vi "DSiam.vi"() -> ()   [LabVIEW 2011]
uses:
  SIAM/SIAM_command.ctl
  SIAM/SIAM-send.ctl
panel:
  out "notifier name":string
  out "send error":errorcluster
  out "value send":dbl
  out "Running":bool
  in  "Scales and Tickets":T1(array[cluster])=[{"ticketID"=514, "Queue/Variable"=FALSE, "name"="stage.z", "Scale"=2e-09, "Offset(HWunits)"=0.0}]
  out "address":string="10.153.70.38"
  out "remote port or service name":u16=3
  out "connect error":errorcluster
  out "Return":i32[](array[numeric]) format="%.0x"
  out "recieve error":errorcluster
  out "Connected":bool
  # "to do\nlimits?\nclosed loop über DSmartmove oder DSIAM oder Smartconnect?\n...\n...\n\n.. Objektivwechsel..."
  # "1122=normal exit"
  # "66=normal exit"
  # "bisher üblich steps/units!!! Logischer für filter!"
  # "becarefull with queues, if there is no reciever it is a memory leak"
  # "ticket  is also inside SIAM-TMSI.vi"
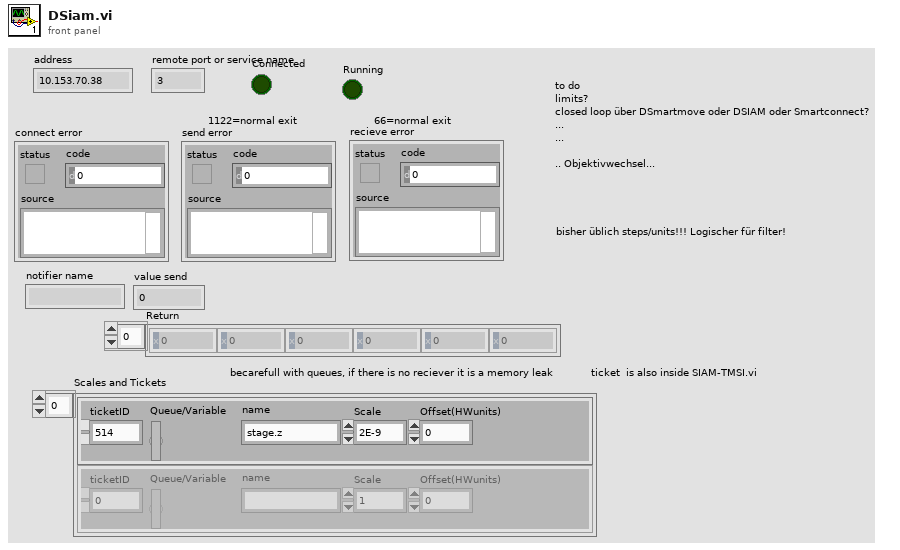
[diagram p1: front panel]
types:
  T1 = cluster{"ticketID":i32, "Queue/Variable":bool, "name":string, "Scale":dbl, "Offset(HWunits)":dbl}[]
  T2 = enum16{"None/#Datasets", "Clear", "TagValueOf#", "AddValues", "ReadValue", "ChangeValue", "Get all"}
  T3 = cluster{"Scale":dbl, "Offset(HWunits)":dbl, "ticketID":i32}[]
  T4 = typedef "SIAM-send.ctl" = enum16{"validID", "storeID", "enable", "rundirect", "sendlist", "run", "stop", "readRegister", "sendValue", "storeStatus"}
  T5 = enum8{"Ch0", "Ch1", "x-Galvo", "y-Galvo", "z-Focus"}
  T6 = enum16{"Ch0", "Ch1", "x-Galvo", "y-Galvo", "z-Focus"}
  T7 = enum16{"Standard", "Buffered", "CRLF", "Immediate"}
  T8 = typedef "SIAM_command.ctl" = u32
  T9 = cluster{"Delay 10µs":u32, "command":T8, "P0":i32, "P1":i32, "P2":i32, "P3":i32, "P4":i32, "P5-ticket":i32}
  T10 = cluster{"Scale":ext, "Offset(HWunits)":ext, "ticketID":i32}[]
  T11 = cluster{"ticketID":i32, "Queue/Variable":bool, "name":string, "Scale":dbl, "Offset(HWunits)":dbl}
  T12 = cluster{"variables":string[], cluster{"Scale":ext, "Offset(HWunits)":ext, "ticketID":i32}[]}
  T13 = cluster{"default value 2":dbl, "default value 1":dbl}
  T14 = cluster{"Delay 10µs":u32, "command":T8, "P0":i32, "P1":i32, "P2":i32, "P3":i32, "P4":i32, "P5-ticket":i32}[]
  T15 = cluster{"Scale":ext, "Offset(HWunits)":ext, "ticketID":i32}
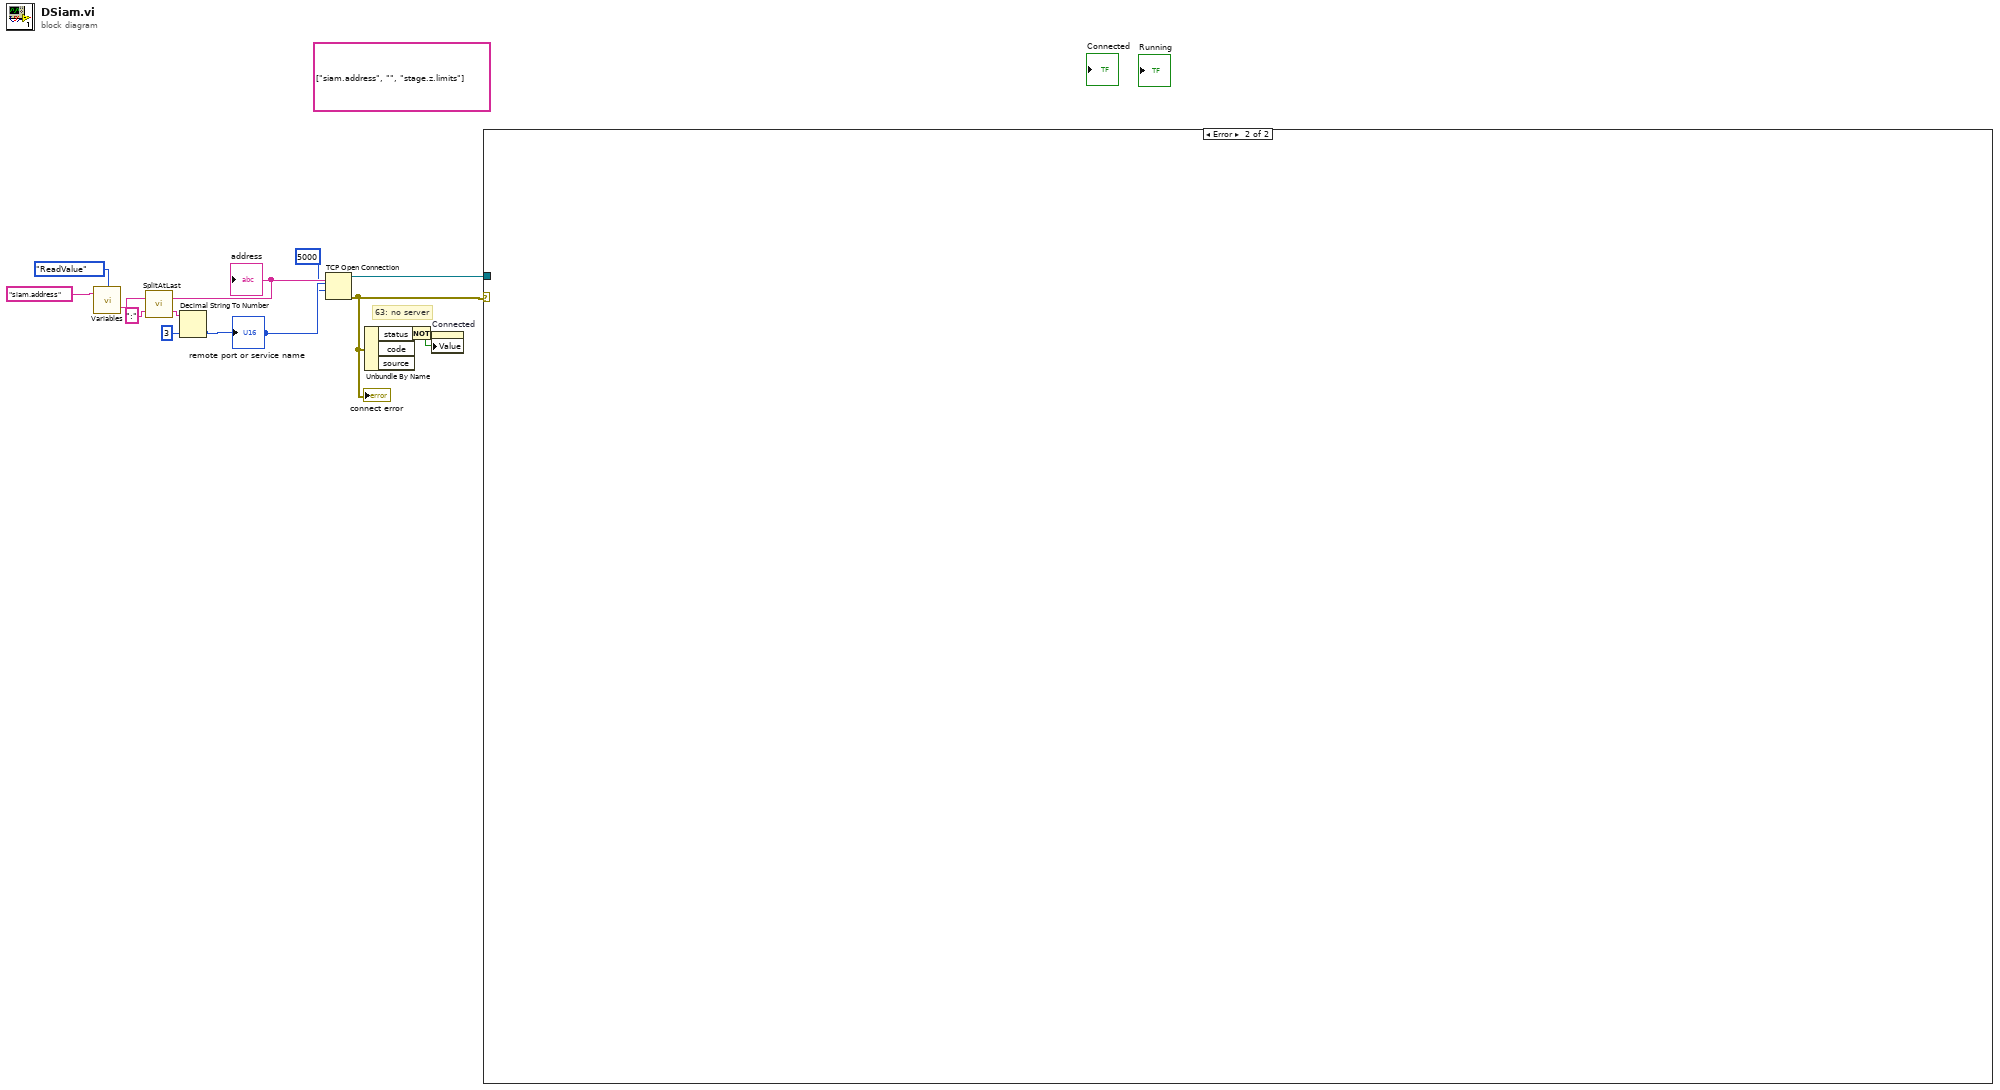
[diagram p0: block diagram]
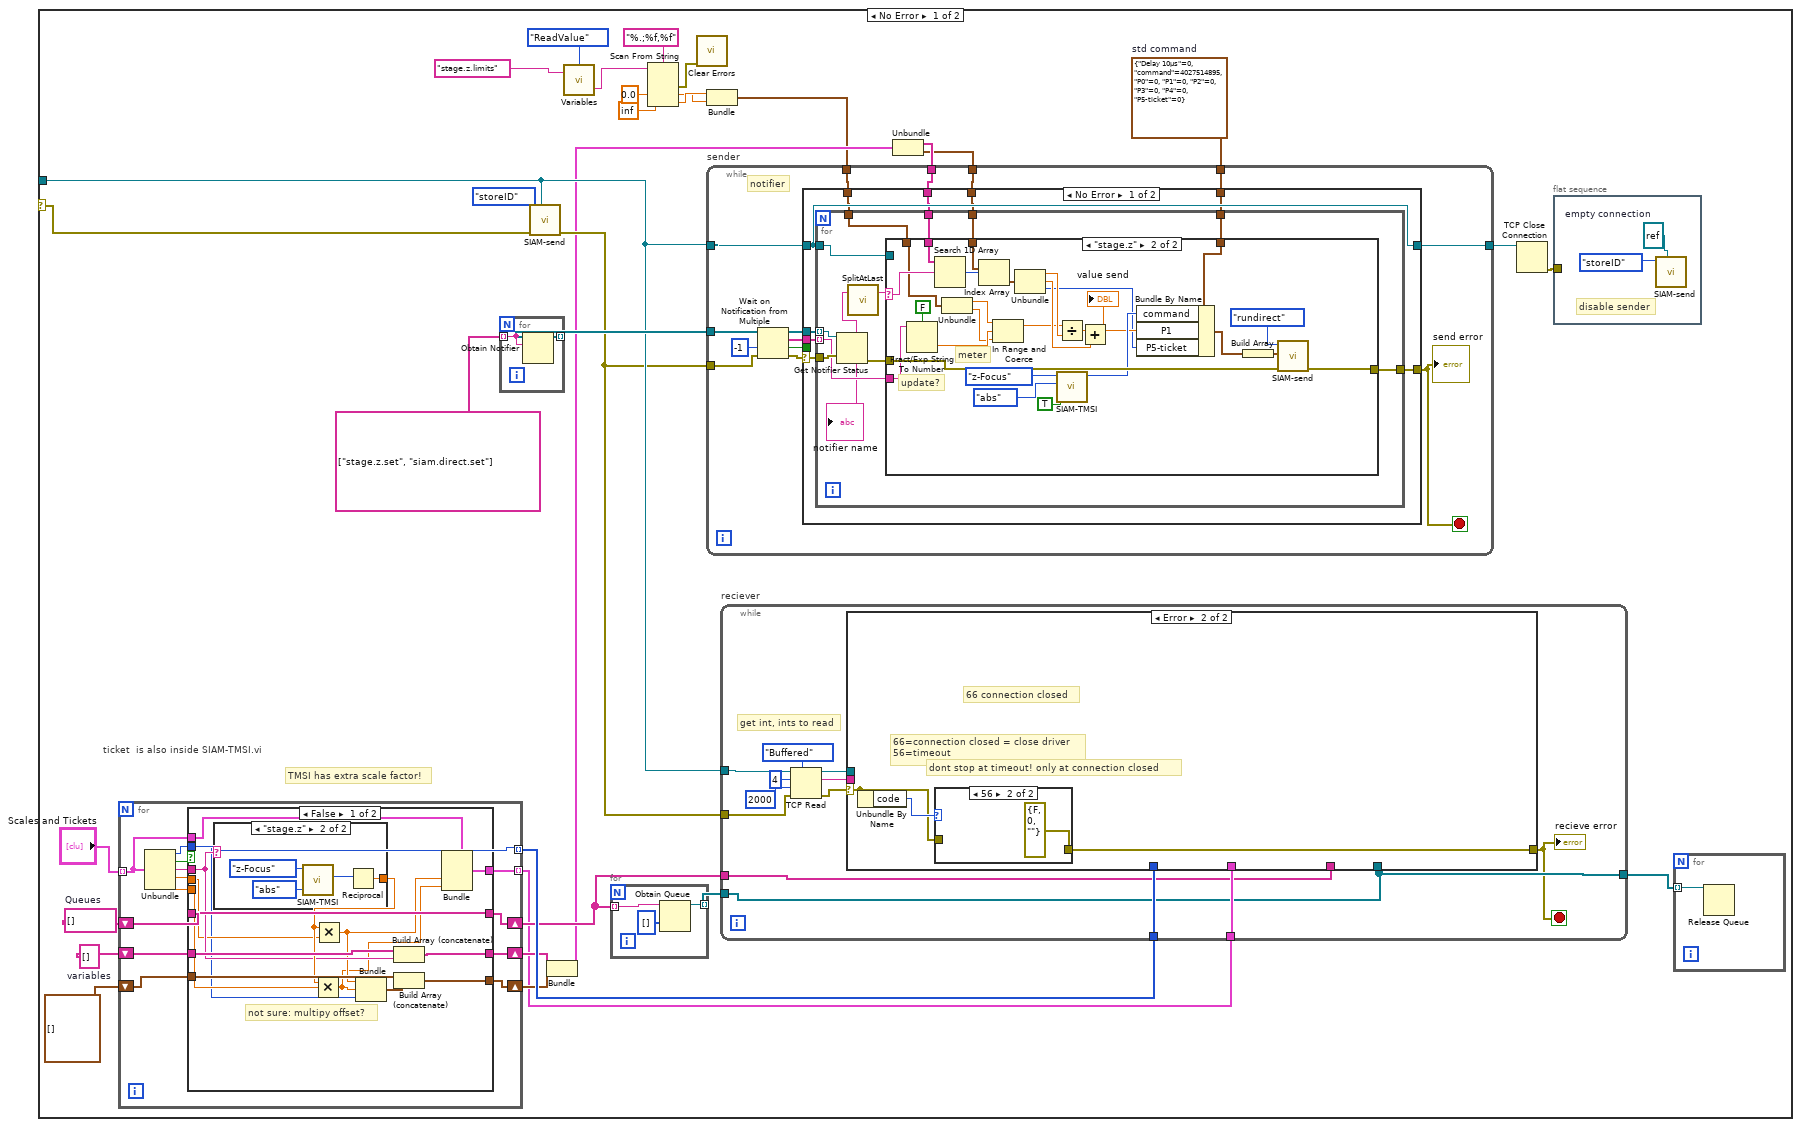
[diagram p2: hidden frame]
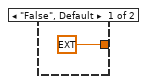
[diagram p3: hidden frame]
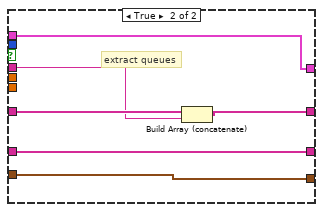
[diagram p4: hidden frame]
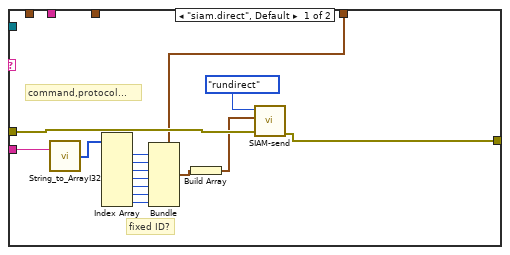
[diagram p5: hidden frame]
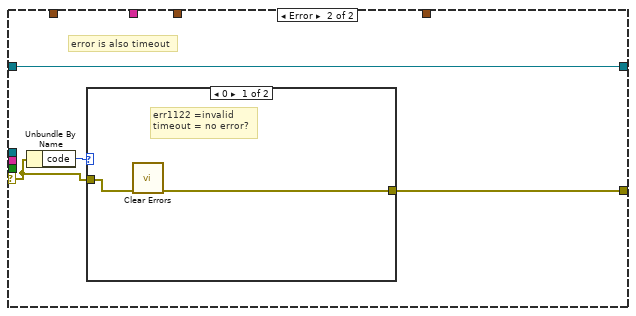
[diagram p6: hidden frame]
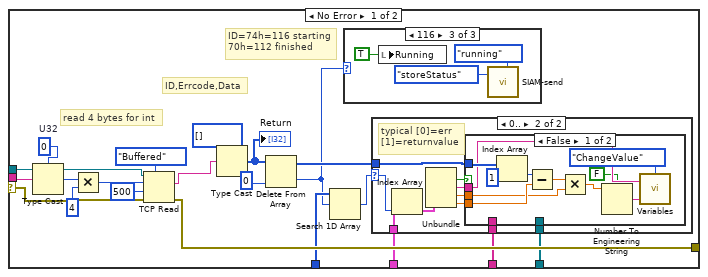
[diagram p8: hidden frame]
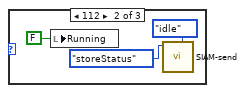
[diagram p10: hidden frame]
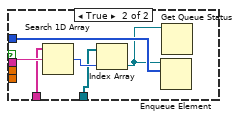
[diagram p12: hidden frame]
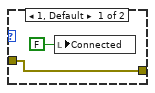
[diagram p13: hidden frame]
diagram:
  (unwired) string[] ["siam.address", "", "stage.z.limits"]
  # "63: no server"
  n1 = call "Variables.vi"("Tag in"="siam.address", "Command"=T2."ReadValue") -> ("value out"=w4:string)  [unwired: 2 in, 1 out]
  n2 = call "SplitAtLast.vi"("search char"=":", "In-String"=w4) -> ("end"=w8:string, "Front (default)"=w9:string)
  "address" <- w9
  n3 = Decimal String To Number(string=w8, default (0L)=3 ("default (0 I32)")) -> (number=w6:i32)  [unwired: 1 in, 1 out]
  "remote port or service name" <- w6
  n4 = TCP Open Connection(address=w9, remote port or service name=w6, timeout ms (60000)=5000) -> (connection ID=w5:refnum<k5>, error out=w2:errorcluster)  [unwired: 1 in, 1 out]
  "connect error" <- w2
  n5 = Unbundle By Name(w2) -> ("status"=w13:bool)  [unwired: 2 out]
  n6 = Not(x=w13) -> (.not. x?=w3:bool)
  n7 = property on="Connected" class="Bool (strict)"("Value"=w3) -> ()  [unwired: 2 in, 2 out]
  n8 = case shown="Error" w2 {
    selector: w2 -> [w14 _]
    tunnel: w5 -> [w38 _]
    frame No Error {
      w34 = string[] []  # variables
      w35 = T9 {"Delay 10µs"=0, "command"=4027514895, "P0"=0, "P1"=0, "P2"=0, "P3"=0, "P4"=0, "P5-ticket"=0}  # std command
      w42 = string[] []  # Queues
      # "ticket  is also inside SIAM-TMSI.vi"
      # "TMSI has extra scale factor!"
      n9 = for {
        tunnel: "Scales and Tickets" -> [w59] mode=indexing
        tunnel: [w54] -> w44 mode=indexing
        shift-right: [w64] -> w39
        shift-left: w42 -> [w65]
        shift-right: [w62] -> w32
        shift-left: w34 -> [w63]
        shift-right: [w60] -> w31
        shift-left: T3 [] -> [w61]
        tunnel: [w53] -> w26 mode=indexing
        n10 = Unbundle(w59) -> ("ticketID"=w54:i32, "Queue/Variable"=w58:bool, "name"=w57:string, "Scale"=w56:dbl, "Offset(HWunits)"=w55:dbl)
        n11 = case shown="False" w58 {
          tunnel: w65 -> [w80 w91]
          tunnel: [w80 w89] -> w64
          tunnel: w57 -> [w73 w90]
          tunnel: w59 -> [w69 w86]
          tunnel: w63 -> [w79 w88]
          tunnel: [w78 w88] -> w62
          tunnel: w61 -> [w77 w87]
          tunnel: [w76 w87] -> w60
          tunnel: w56 -> [w71 _]
          tunnel: w55 -> [w72 _]
          tunnel: w54 -> [w70 _]
          tunnel: [w66 w86] -> w53
          frame False {
            # "not sure: multipy offset?"
            n12 = case shown="\"stage.z\"" w73 {
              tunnel: [ext 1.0 w85] -> w74
              frame "False", Default {
              }
              frame "stage.z" {
                n13 = call "SIAM-TMSI.vi"("Type"=enum8{"acc", "vel", "abs", "offset"}."abs", "Motor"=T5."z-Focus") -> ("Resolution-Factor"=w82:i32)  [unwired: 6 in, 3 out]
                n14 = Reciprocal(x=w82) -> (1/x=w85:dbl)
              }
            }
            n15 = Multiply(x=w74, y=w72) -> (x*y=w67:ext)
            n16 = Multiply(x=w74, y=w71) -> (x*y=w68:ext)
            n17 = Bundle(w68, w67, "ticketID"=w70) -> (w75:cluster{ext, ext, "ticketID":i32})  [unwired: 1 in]
            n18 = Build Array (concatenate)(w79, w73) -> (w78:string[])
            n19 = Build Array (concatenate)(w77, w75) -> (w76:T10)
            n20 = Bundle(cluster=w69, "Scale"=w68, "Offset(HWunits)"=w67) -> (w66:T11)  [unwired: 3 in]
          }
          frame True {
            # "extract queues"
            n21 = Build Array (concatenate)(w91, w90) -> (w89:string[])
          }
        }
      }
      n22 = for {
        tunnel: [w93] -> w46 mode=indexing
        tunnel: string[] ["stage.z.set", "siam.direct.set"] -> [w92] mode=indexing
        n23 = Obtain Notifier(name (unnamed)=w92, notification data type=w92) -> (notifier out=w93:refnum<notifier>)  [unwired: 2 in, 2 out]
      }
      n24 = call "SIAM-send.vi"("connection ID"=w38, "error in (no error)"=w14, "command"=SIAM-send."storeID") -> ("error out"=w36:errorcluster)  [unwired: 7 in, 1 out]
      n25 = Bundle("variables"=w32, w31) -> (w30:T12)  [unwired: 1 in]
      n26 = call "Variables.vi"("Tag in"="stage.z.limits", "Command"=T2."ReadValue") -> ("value out"=w23:string)  [unwired: 1 in, 2 out]
      n27 = for {
        tunnel: w39 -> [w52] mode=indexing
        tunnel: [w51] -> w41 mode=indexing
        n28 = Obtain Queue(name (unnamed)=w52, element data type=i32[] []) -> (queue out=w51:refnum<queue>)  [unwired: 3 in, 2 out]
      }
      n29 = Scan From String(format string="%.;%f,%f", input string=w23, default 1=0.0 ("default value 1"), default 2=inf ("default value 2")) -> (error out=w17:errorcluster, output 1=w18:dbl, output 2=w19:dbl)  [unwired: 2 in, 2 out]
      n30 = call <vilib>:"Clear Errors.vi"("error in (no error)"=w17) -> ()  [unwired: 7 out]
      n31 = Bundle("default value 2"=w19, "default value 1"=w18) -> (w16:T13)  [unwired: 1 out]
      n32 = while "reciever" {
        tunnel: w38 -> [w190]
        tunnel: w44 -> [w183]
        tunnel: w26 -> [w182]
        tunnel: w41 -> [w181]
        tunnel: [w181] -> w40
        tunnel: w39 -> [w180]
        tunnel: w36 -> [w178]
        stop <- w179 stop-if-true
        # "get int, ints to read"
        n33 = TCP Read(connection ID=w190, bytes to read=4, error in (no error)=w178, 7:T7."Buffered" ("mode (standard)"), 9:2000 ("timeout ms (25000)")) -> (connection ID out=w186:refnum<k5>, data out=w187:string, error out=w184:errorcluster)
        n34 = case shown="Error" w184 {
          selector: w184 -> [w207 w245]
          tunnel: w187 -> [w211 _]
          tunnel: w186 -> [w208 _]
          tunnel: [w202 w246] -> w179
          tunnel: w183 -> [w197 _]
          tunnel: w182 -> [w196 _]
          tunnel: w181 -> [w192 _]
          tunnel: w180 -> [w191 _]
          frame No Error {
            w210 = u32 0  # U32
            # "ID=74h=116 starting\n70h=112 finished"
            # "read 4 bytes for int"
            # "ID,Errcode,Data"
            n35 = Type Cast(type=w210, x=w211) -> (*(type *) &x=w205:u32)
            n36 = Multiply(x=w205, y=u32 4) -> (x*y=w203:u32)
            n37 = TCP Read(connection ID=w208, bytes to read=w203, error in (no error)=w207, 7:T7."Buffered" ("mode (standard)"), 9:500 ("timeout ms (25000)")) -> (data out=w201:string, error out=w202:errorcluster)  [unwired: 1 out]
            n38 = Type Cast(type=i32[] [], x=w201) -> (*(type *) &x=w199:i32[])
            "Return" <- w199
            n39 = Delete From Array(array=w199, index=0) -> (deleted portion=w193:i32, array with subset deleted=w194:i32[])  [unwired: 1 in]
            n40 = Search 1D Array(1D array=w197, element=w193) -> (index of element=w195:i32)  [unwired: 1 in]
            n41 = case shown="116" w193 {
              frame 0, Default {
              }
              frame 112 {
                n42 = local write "Running"(FALSE ("Running")) -> ()
                n43 = call "SIAM-send.vi"("Value"=enum16{"unknown", "idle", "running", ""}."idle" ("Status"), "command"=SIAM-send."storeStatus") -> ()  [unwired: 8 in, 2 out]
              }
              frame 116 {
                n44 = local write "Running"(TRUE ("Running")) -> ()
                n45 = call "SIAM-send.vi"("Value"=enum16{"unknown", "idle", "running", ""}."running" ("Status"), "command"=SIAM-send."storeStatus") -> ()  [unwired: 8 in, 2 out]
              }
            }
            n46 = case shown="0.." w195 {
              selector: w195 -> [_ w226]
              tunnel: w196 -> [_ w227]
              tunnel: w194 -> [_ w223]
              tunnel: w192 -> [_ w219]
              tunnel: w191 -> [_ w218]
              frame -1, Default {
                # "no rule"
              }
              frame 0.. {
                # "typical [0]=err\n[1]=returnvalue"
                n47 = Index Array(array=w227, index=w226) -> (element=w225:T11)
                n48 = Unbundle(w225) -> ("Queue/Variable"=w224:bool, "name"=w220:string, "Scale"=w221:dbl, "Offset(HWunits)"=w222:dbl)  [unwired: 1 out]
                n49 = case shown="False" w224 {
                  tunnel: w223 -> [w238 w240]
                  tunnel: w222 -> [w236 _]
                  tunnel: w221 -> [w234 _]
                  tunnel: w220 -> [w233 w244]
                  tunnel: w219 -> [_ w241]
                  tunnel: w218 -> [_ w243]
                  frame False {
                    n50 = Index Array(array=w238, index=1) -> (element=w237:i32)
                    n51 = Subtract(x=w237, y=w236) -> (x-y=w235:dbl)
                    n52 = Multiply(x=w235, y=w234) -> (x*y=w231:dbl)
                    n53 = Number To Engineering String(1:FALSE ("use system decimal point (T)"), 4:w231) -> (0:w230:string)  [unwired: 2 out]
                    n54 = call "Variables.vi"("value"=w230, "Tag in"=w233, "Command"=T2."ChangeValue") -> ()  [unwired: 1 in, 2 out]
                  }
                  frame True {
                    n55 = Search 1D Array(1D array=w243, element=w244) -> (index of element=w242:i32)  [unwired: 1 in]
                    n56 = Index Array(array=w241, index=w242) -> (element=w239:refnum<queue>)
                    n57 = Enqueue Element(queue=w239, element=w240) -> ()  [unwired: 2 in, 3 out]
                    n58 = Get Queue Status(queue=w239) -> ()  [unwired: 2 in, 8 out]
                  }
                }
              }
            }
          }
          frame Error {
            # "66 connection closed"
            # "dont stop at timeout! only at connection closed"
            # "66=connection closed = close driver\n56=timeout"
            n59 = Unbundle By Name(w245) -> ("code"=w247:i32)
            n60 = case shown="56" w247 {
              tunnel: [w249 errorcluster {"status"=FALSE, "code"=0, "source"=""} ("error out")] -> w246
              tunnel: w245 -> [w249 _]
              frame 1, Default {
                n61 = local write "Connected"(FALSE ("Connected")) -> ()
              }
              frame 56 {
              }
            }
          }
        }
        "recieve error" <- w179
      }
      n62 = Unbundle(w30) -> ("variables"=w29:string[], w28:T10)
      n63 = while "sender" {
        tunnel: w38 -> [w105]
        tunnel: w46 -> [w104]
        tunnel: [w102] -> w43
        tunnel: w36 -> [w101]
        tunnel: w35 -> [w97]
        tunnel: w29 -> [w96]
        tunnel: w28 -> [w95]
        tunnel: w16 -> [w94]
        stop <- w98 stop-if-true
        # "notifier"
        n64 = Wait on Notification from Multiple(0:w104, 2:-1 ("timeout in ms (-1)"), 3:w101) -> (8:w107:refnum<notifier>[], 9:w106:string[], 10:w99:bool, 11:w100:errorcluster)  [unwired: 1 in]
        n65 = case shown="No Error" w100 {
          selector: w100 -> [w113 w171]
          tunnel: w107 -> [w116 _]
          tunnel: w106 -> [w115 _]
          tunnel: w105 -> [w114 w174]
          tunnel: [w114 w174] -> w102
          tunnel: w99 -> [_ _]
          tunnel: [w112 w173] -> w98
          tunnel: w97 -> [w111 _]
          tunnel: w96 -> [w110 _]
          tunnel: w95 -> [w109 _]
          tunnel: w94 -> [w108 _]
          frame No Error {
            n66 = for {
              tunnel: w116 -> [w127] mode=indexing
              tunnel: w115 -> [w126] mode=indexing
              tunnel: w114 -> [w125]
              tunnel: w113 -> [w128]
              tunnel: [w124] -> w112
              tunnel: w111 -> [w122]
              tunnel: w110 -> [w121]
              tunnel: w109 -> [w120]
              tunnel: w108 -> [w117]
              n67 = Get Notifier Status(notifier=w127, error in (no error)=w128) -> (notifier name=w119:string, error out=w123:errorcluster)  [unwired: 3 out]
              "notifier name" <- w119
              n68 = call "SplitAtLast.vi"("In-String"=w119) -> ("Front (default)"=w118:string)  [unwired: 1 in, 1 out]
              n69 = case shown="\"stage.z\"" w118 {
                selector: w118 -> [_ w165]
                tunnel: w126 -> [w140 w169]
                tunnel: w125 -> [_ _]
                tunnel: [w142 w150] -> w124
                tunnel: w123 -> [w141 w170]
                tunnel: w122 -> [w138 w159]
                tunnel: w121 -> [_ w164]
                tunnel: w120 -> [_ w162]
                tunnel: w117 -> [_ w145]
                frame "siam.direct", Default {
                  # "fixed ID?"
                  # "command,protocol..."
                  n70 = call "String_to_ArrayI32.vi"("String"=w140) -> ("ArrayI32"=w139:i32[])  [unwired: 1 in]
                  n71 = Index Array(array=w139) -> (element #1=w137:i32, element #2=w136:i32, element #3=w135:i32, element #4=w134:i32, element #5=w133:i32, element #6=w132:i32, element #7=w131:i32)  [unwired: 7 in]
                  n72 = Bundle(cluster=w138, "command"=w137, "P0"=w136, "P1"=w135, "P2"=w134, "P3"=w133, "P4"=w132, "P5-ticket"=w131) -> (w130:T9)  [unwired: 1 in]
                  n73 = Build Array(w130) -> (w129:T14)
                  n74 = call "SIAM-send.vi"("error in (no error)"=w141, "Script"=w129, "command"=SIAM-send."rundirect") -> ("error out"=w142:errorcluster)  [unwired: 7 in, 1 out]
                }
                frame "stage.z" {
                  # "meter"
                  # "update?"
                  n75 = Fract/Exp String To Number(use system decimal point (T)=FALSE, string=w169) -> (number=w148:dbl)  [unwired: 2 in, 1 out]
                  n76 = Search 1D Array(1D array=w164, element=w165) -> (index of element=w163:i32)  [unwired: 1 in]
                  n77 = Unbundle(w145) -> ("default value 2"=w146:dbl, "default value 1"=w147:dbl)
                  n78 = Index Array(array=w162, index=w163) -> (element=w161:T15)
                  n79 = In Range and Coerce(upper limit=w146, x=w148, lower limit=w147) -> (coerced(x)=w144:dbl)  [unwired: 1 out]
                  n80 = Unbundle(w161) -> ("Scale"=w157:ext, "Offset(HWunits)"=w156:ext, "ticketID"=w149:i32)
                  n81 = Divide(x=w144, y=w157) -> (x/y=w160:ext)
                  n82 = call "SIAM-TMSI.vi"("use ticket"=TRUE, "Type"=enum8{"acc", "vel", "abs", "offset"}."abs", "Motor"=T6."z-Focus") -> ("command"=w153:T8)  [unwired: 5 in, 3 out]
                  n83 = Add(x=w160, y=w156) -> (x+y=w152:ext)
                  "value send" <- w152
                  n84 = Bundle By Name(cluster=w159, "command"=w153, "P1"=w152, "P5-ticket"=w149) -> (w167:T9)
                  n85 = Build Array(w167) -> (w166:T14)
                  n86 = call "SIAM-send.vi"("error in (no error)"=w170, "Script"=w166, "command"=SIAM-send."rundirect") -> ("error out"=w150:errorcluster)  [unwired: 7 in, 1 out]
                }
              }
            }
          }
          frame Error {
            # "error is also timeout"
            n87 = Unbundle By Name(w171) -> ("code"=w172:i32)
            n88 = case shown="0" w172 {
              tunnel: [w176 w177] -> w173
              tunnel: w171 -> [w175 w177]
              frame 0 {
                # "err1122 =invalid\ntimeout = no error?"
                n89 = call <vilib>:"Clear Errors.vi"("error in (no error)"=w175) -> ("error out"=w176:errorcluster)  [unwired: 6 in]
              }
              frame 1122, Default {
                # "close notifier = stop driver"
              }
            }
          }
        }
        "send error" <- w98
      }
      n90 = TCP Close Connection(connection ID=w43) -> (error out=w15:errorcluster)  [unwired: 2 in, 1 out]
      n91 = flat-sequence {
        tunnel: w15 -> [_]
        frame #0 {
          w47 = refnum<k5> refnum  # empty connection
          # "disable sender"
          n92 = call "SIAM-send.vi"("connection ID"=w47, "command"=SIAM-send."storeID") -> ()  [unwired: 8 in, 2 out]
        }
      }
      n93 = for {
        tunnel: w40 -> [w49] mode=indexing
        n94 = Release Queue(queue=w49) -> ()  [unwired: 2 in, 3 out]
      }
    }
    frame Error {
    }
  }
